vi "Main.vi"(7 "Action":T2=enum."Close", 8 "Error In":errorcluster, 11 "Input":variant) -> (0 "Error Out":errorcluster, 3 "Output":variant)   [LabVIEW 2018, in "Database.lvlib"]
doc: "Action Engine for the module. This private VI is wrapped for the API."
uses:
  Database.lvlib
  Action.ctl
  <vilib>/addons/database/Connection.llb/Conn Properties.ctl
  <vilib>/addons/database/Connection.llb/Conn ObjectReference.ctl
  <vilib>/addons/database/Connection.llb/DB Tools Open Connec (Path).vi
  <vilib>/addons/database/Connection.llb/Conn Execute.vi
  <vilib>/addons/database/Recordset.llb/Rec Fetch Recordset Data (R).vi
  <vilib>/addons/database/Recordset.llb/Rec Destroy - Connection.vi
  <vilib>/Utility/error.llb/Error Cluster From Error Code.vi
  <vilib>/ErrorRing/Error Ring.xnode
  <vilib>/addons/database/NI_Database_API.lvlib
  <vilib>/addons/database/Connection.llb/Conn Get Properties.vi
panel:
  out "connection properties":T1
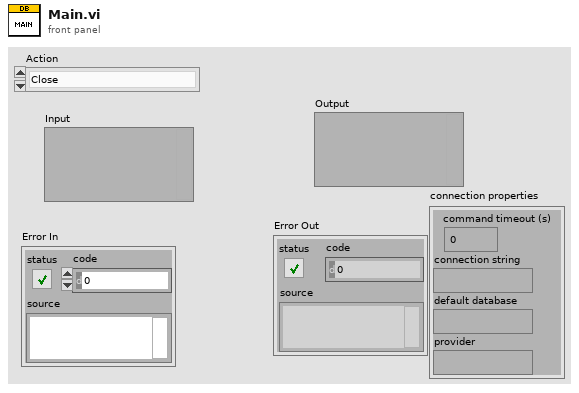
[diagram p1: front panel]
types:
  T1 = typedef "NI_Database_API.lvlib/Conn Properties.ctl" = cluster{"command timeout (s)":i32, "connection string":string, "default database":string, "provider":string}
  T2 = typedef "Database.lvlib/Action.ctl" = enum16{"Init", "List Tables", "List Columns", "Query", "Close"}
  T3 = typedef "NI_Database_API.lvlib/Conn ObjectReference.ctl" = refnum<k1>
  T4 = typedef "NI_Database_API.lvlib/DB Tools DataTypes.ctl" = enum16{"String", "Long (I32)", "Single (SGL)", "Double (DBL)", "Date/Time", "Binary"}
  T5 = cluster{"name":string, "database data type":T4, "defined size":i32}[]
  T6 = cluster{"column information":cluster{"name":string, "database data type":T4, "defined size":i32}[], "columns":string[]}
  T7 = typedef "NI_Database_API.lvlib/Rec ObjectReference.ctl" = refnum<k1>
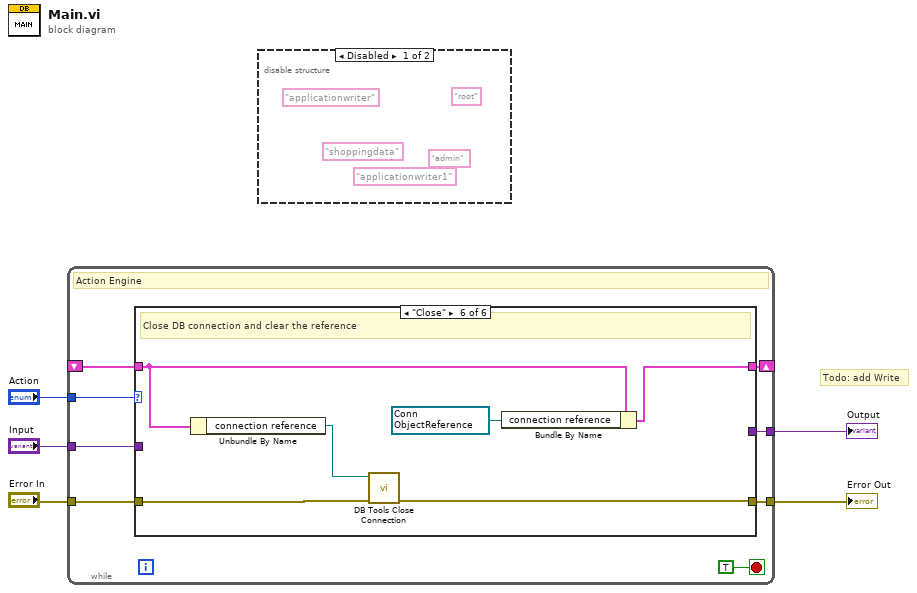
[diagram p0: block diagram]
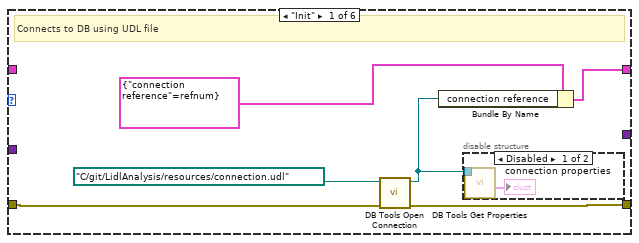
[diagram p3: hidden frame]
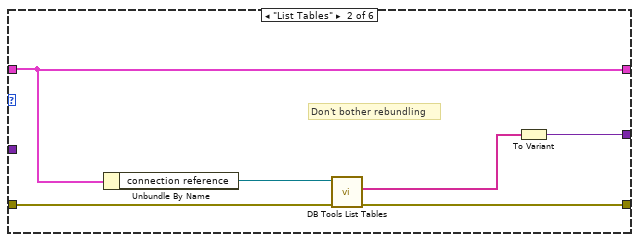
[diagram p5: hidden frame]
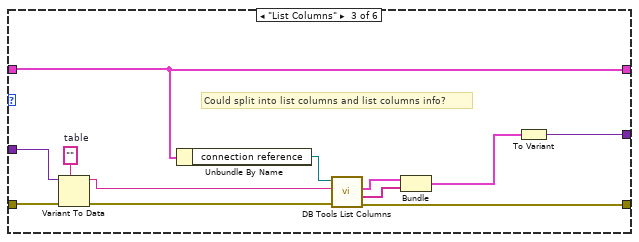
[diagram p6: hidden frame]
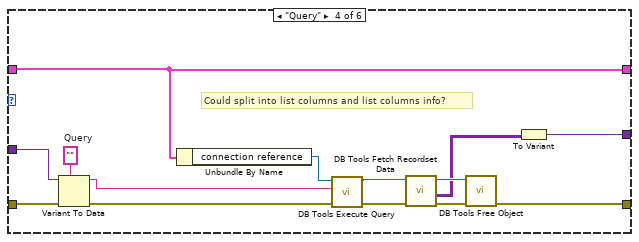
[diagram p7: hidden frame]
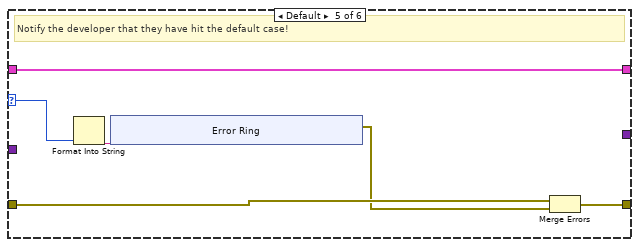
[diagram p8: hidden frame]
diagram:
  # "Todo: add Write"
  n1 = while {
    tunnel: "Error In" -> [w11]
    tunnel: [w12] -> w4
    tunnel: "Action" -> [w10]
    shift-right: [w9] -> _
    shift-left: _ -> [w8]
    tunnel: [w7] -> w2
    tunnel: "Input" -> [w6]
    stop <- TRUE stop-if-true
    # "Action Engine"
    n2 = case shown="\"Close\"" w10 {
      selector: w10 -> [_ _ _ _ w55 _]
      tunnel: [w18 w25 w37 w40 w59 w71] -> w12
      tunnel: w11 -> [w17 w24 w34 w49 w58 w72]
      tunnel: [w15 w27 w39 w53 w54 w68] -> w9
      tunnel: w8 -> [_ w27 w39 w53 w54 w69]
      tunnel: [_ w22 w36 w51 _ _] -> w7
      tunnel: w6 -> [_ _ w33 w48 _ _]
      frame "Init" {
        # "Connects to DB using UDL file"
        n3 = call-poly <vilib>:"DB Tools Open Connection.vi"("error in (no error)"=w17, "connection information"=path "C:/git/LidlAnalysis/resources/connection.udl") -> ("error out"=w18:errorcluster, "connection reference"=w14:T3)  [unwired: 6 in]
        n4 = Bundle By Name(cluster=cluster{"connection reference":T3} {"connection reference"=refnum}, "connection reference"=w14) -> (w15:cluster{"connection reference":T3})
        n5 = disable-structure shown="Disabled" {
          disable-tunnel: w14 -> [w21 _]
          frame Disabled {
            n6 = call-poly <vilib>:"DB Tools Get Properties.vi"("connection reference"=w21) -> ("connection properties"=→"connection properties":T1)  [unwired: 4 in, 2 out]
          }
          frame Enabled {
          }
        }
      }
      frame "List Tables" {
        # "Don't bother rebundling"
        n7 = Unbundle By Name(w27) -> ("connection reference"=w26:T3)
        n8 = call <vilib>:"DB Tools List Tables.vi"("error in (no error)"=w24, "connection reference"=w26) -> ("error out"=w25:errorcluster, "tables"=w23:string[])  [unwired: 3 in, 1 out]
        n9 = To Variant(anything=w23) -> (Variant=w22:variant)
      }
      frame "List Columns" {
        w32 = ""  # table
        # "Could split into list columns and list columns info?"
        n10 = Variant To Data(error in=w34, type=w32, Variant=w33) -> (data=w31:string, error out=w35:errorcluster)
        n11 = Unbundle By Name(w39) -> ("connection reference"=w38:T3)
        n12 = call <vilib>:"DB Tools List Columns.vi"("error in (no error)"=w35, "table"=w31, "connection reference"=w38) -> ("error out"=w37:errorcluster, "columns"=w30:string[], "column information"=w29:T5)  [unwired: 1 in, 1 out]
        n13 = Bundle("column information"=w29, "columns"=w30) -> (w28:T6)  [unwired: 1 in]
        n14 = To Variant(anything=w28) -> (Variant=w36:variant)
      }
      frame "Query" {
        w47 = ""  # Query
        # "Could split into list columns and list columns info?"
        n15 = Variant To Data(error in=w49, type=w47, Variant=w48) -> (data=w46:string, error out=w50:errorcluster)
        n16 = Unbundle By Name(w53) -> ("connection reference"=w52:T3)
        n17 = call-poly <vilib>:"DB Tools Execute Query.vi"("error in (no error)"=w50, "SQL query"=w46, "connection reference"=w52) -> ("error out"=w45:errorcluster, "recordset reference"=w44:T7)  [unwired: 5 in]
        n18 = call-poly <vilib>:"DB Tools Fetch Recordset Data.vi"("error in (no error)"=w45, "recordset reference"=w44) -> ("error out"=w43:errorcluster, "recordset data"=w41:variant[][], "recordset reference out"=w42:T7)  [unwired: 3 in]
        n19 = call-poly <vilib>:"DB Tools Free Object.vi"("error in (no error)"=w43, "recordset reference"=w42) -> ("error out"=w40:errorcluster)  [unwired: 8 in, 1 out]
        n20 = To Variant(anything=w41) -> (Variant=w51:variant)
      }
      frame Default {
        # "Notify the developer that they have hit the default case!"
        n21 = Format Into String(w55) -> (resulting string=w56:string)  [unwired: 3 in, 1 out]
        n22 = xnode "Error Ring"("parameter 0"=w56) -> ("error out"=w57:errorcluster)
        n23 = Merge Errors(w58, w57) -> (w59:errorcluster)
      }
      frame "Close" {
        w67 = T3 refnum items=["Connection"] ("connection reference")
        # "Close DB connection and clear the reference"
        n24 = Unbundle By Name(w69) -> ("connection reference"=w70:T3)
        n25 = call <vilib>:"DB Tools Close Connection.vi"("error in (no error)"=w72, "connection reference"=w70) -> ("error out"=w71:errorcluster)  [unwired: 5 in]
        n26 = Bundle By Name(cluster=w69, "connection reference"=w67) -> (w68:cluster{"connection reference":T3})
      }
    }
  }
  "Error Out" <- w4
  "Output" <- w2
  n27 = disable-structure shown="Disabled" {
    frame Disabled {
      (unwired) "root" ("userID")
      (unwired) "applicationwriter" ("userID")
      (unwired) "admin" ("password")
      (unwired) "shoppingdata" ("userID")
      (unwired) "applicationwriter1" ("userID")
    }
    frame Enabled {
    }
  }
